vi "Bessel Function Yv.vi"(2 "v":dbl format="%.2f", 3 "x":dbl format="%.2f") -> (1 "Yv(x)":dbl format="%.2f")   [LabVIEW 2020, in "NI_Gmath.lvlib"]
doc: "Computes the Bessel function of the second kind, also known as the Neumann function."
uses:
  <vilib>/gmath/NI_Gmath.lvlib
  <resource>/lvanlys.dll
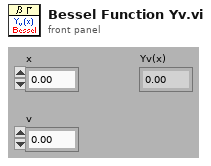
[diagram p1: front panel]
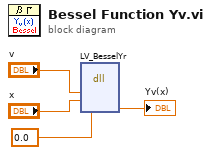
[diagram p0: block diagram]
diagram:
  n1 = dll-call lib="e:/builds/penguin/labview/branches/2020/dev/dist/resource/lvanlys.*" fn="LV_BesselYr"("v"="v", "x"="x", "Yv(x)"=0.0 ("Jr")) -> ("Yv(x)"=→"Yv(x)":dbl)  [unwired: 6 in, 2 out]
